vi "WriteUShortSpectrumAttribute.vi"(2 "value":u16[](array[numeric]), 3 "attribute name":string, 4 "device name":string) -> (0 "error stack":string[](array[string]), 1 "success":bool)   [LabVIEW 2014, in "tango.lvlib"]
uses:
  tango.lvlib
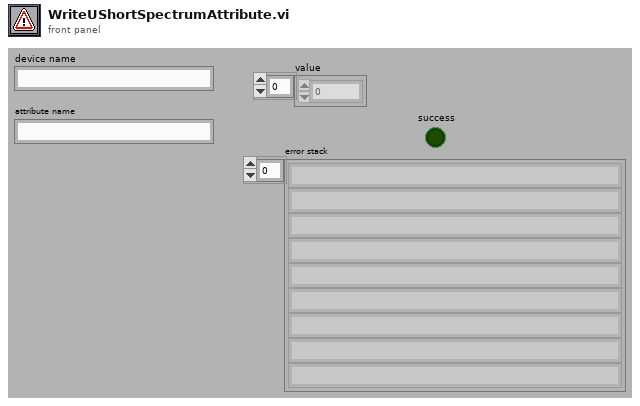
[diagram p1: front panel]
types:
  T1 = cluster{"device name":string, "attribute name":string, "quality value":i16, "quality string":string, "timestamp":dbl, "dim. x":i32, "dim. y":i32, "value":u8[], "error code":i32, "error stack":string[], "data type":u16}
  T2 = cluster{"device name":string, "attribute name":string, "quality value":i16, "quality string":string, "timestamp":dbl, "dim. x":i32, "dim. y":i32, "value":u8[], "error code":i32, "error stack":string[], "data type":u16}[]
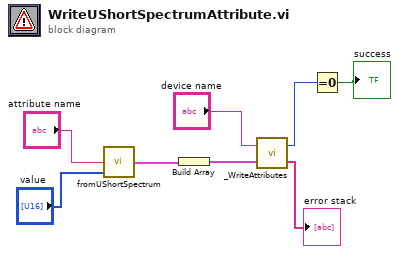
[diagram p0: block diagram]
diagram:
  n1 = call "fromUShortSpectrum.vi"("value"="value", "attribute name"="attribute name") -> ("attribute value"=w5:T1)  [unwired: 1 in]
  n2 = Build Array(w5) -> (w7:T2)
  n3 = call "_WriteAttributes.vi"("attribute Values"=w7, "device name"="device name") -> ("error stack"=→"error stack":string[], "error code"=w2:i32)
  n4 = Equal To 0?(x=w2) -> (x = 0?=→"success":bool)
